vi "TimeToString.vi"(1 "Time Stamp Control":timestamp) -> (0 "result string":string)   [LabVIEW 2017]
panel:
  # "02-MAR-16 17:03:42.529975"
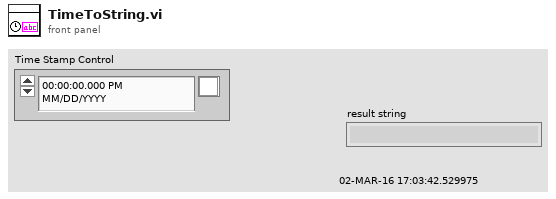
[diagram p1: front panel]
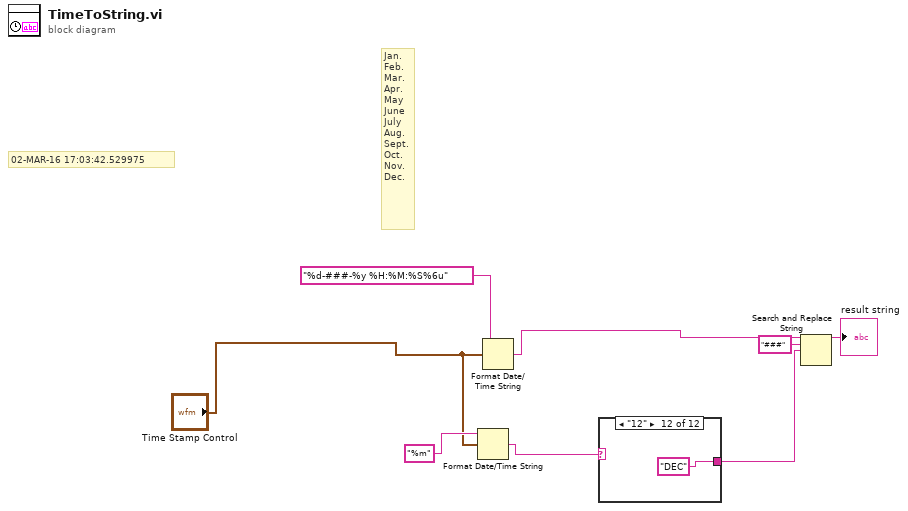
[diagram p0: block diagram]
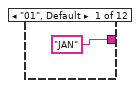
[diagram p2: hidden frame]
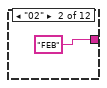
[diagram p3: hidden frame]
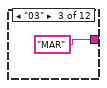
[diagram p4: hidden frame]
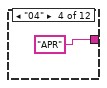
[diagram p5: hidden frame]
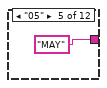
[diagram p6: hidden frame]
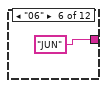
[diagram p7: hidden frame]
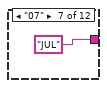
[diagram p8: hidden frame]
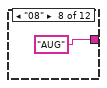
[diagram p9: hidden frame]
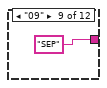
[diagram p10: hidden frame]
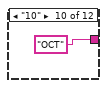
[diagram p11: hidden frame]
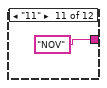
[diagram p12: hidden frame]
diagram:
  # "Jan.\nFeb. \nMar.\nApr.\nMay \nJune\nJuly\nAug.\nSept.\nOct. \nNov.\nDec."
  # "02-MAR-16 17:03:42.529975"
  n1 = Format Date/Time String(time format string (%c)="%m", seconds (now)="Time Stamp Control") -> (date/time string=w8:string)  [unwired: 1 in]
  n2 = Format Date/Time String(time format string (%c)="%d-###-%y %H:%M:%S%6u", seconds (now)="Time Stamp Control") -> (date/time string=w7:string)  [unwired: 1 in]
  n3 = case shown="\"12\"" w8 {
    tunnel: ["JAN" "FEB" "MAR" "APR" "MAY" "JUN" "JUL" "AUG" "SEP" "OCT" "NOV" "DEC"] -> w5
    frame "01", Default {
    }
    frame "02" {
    }
    frame "03" {
    }
    frame "04" {
    }
    frame "05" {
    }
    frame "06" {
    }
    frame "07" {
    }
    frame "08" {
    }
    frame "09" {
    }
    frame "10" {
    }
    frame "11" {
    }
    frame "12" {
    }
  }
  n4 = Search and Replace String(input string=w7, search string="###", replace string=w5) -> (result string=→"result string":string)  [unwired: 5 in, 3 out]
